vi "GE 5565PIORC.Memory.Deallocate Block.vi"(8 "error in (no error)":errorcluster, 10 "Block Descriptor":T1 {"next descriptor ptr" format="%08x"; "data size" format="%08x"; "data ptr (upper)" format="%08x"; "data ptr (lower)" format="%08x"; "descriptor ptr (aligned)" format="%08x"; "descriptor size" format="%08x"; "descriptor ptr (VISA)" format="%08x"}, 11 "GE 5565PIORC in":refnum<class "GE 5565PIORC.lvclass">) -> (0 "error out":errorcluster, 3 "GE 5565PIORC out":refnum<class "GE 5565PIORC.lvclass">)   [LabVIEW 2016, in "GE 5565PIORC.lvclass"]
uses:
  GE 5565PIORC.lvclass
  Typedefs/GE 5565PIORC.Typdef.DMA Block Descriptor.ctl
  GE 5565PIORC.lvclass/GE 5565PIORC.ctl
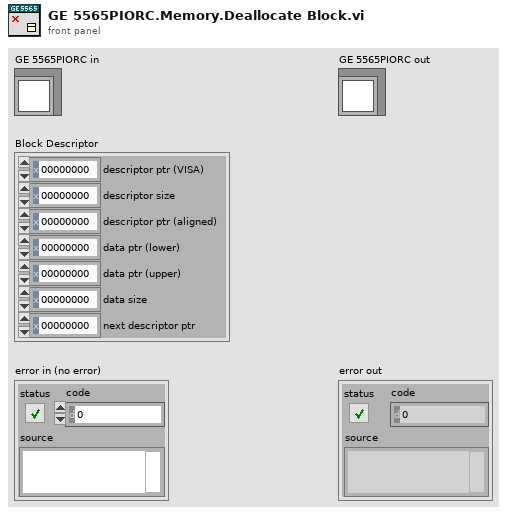
[diagram p1: front panel]
types:
  T1 = typedef "GE 5565PIORC.lvclass/GE 5565PIORC.Typdef.DMA Block Descriptor.ctl" = cluster{"descriptor ptr (VISA)":u32, "descriptor size":u32, "descriptor ptr (aligned)":u32, "data ptr (lower)":u32, "data ptr (upper)":u32, "data size":u32, "next descriptor ptr":u32}
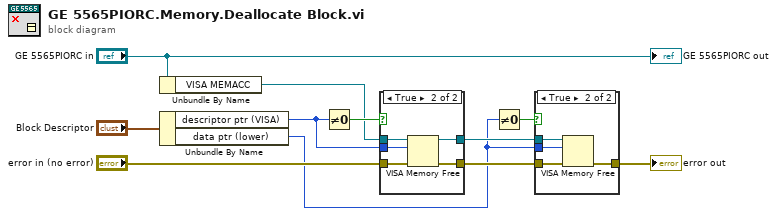
[diagram p0: block diagram]
diagram:
  n1 = Unbundle By Name("GE 5565PIORC in") -> ("VISA MEMACC"=w9:refnum<visa-resource-name>)
  n2 = Unbundle By Name("Block Descriptor") -> ("descriptor ptr (VISA)"=w11:u32, "data ptr (lower)"=w1:u32)
  n3 = Not Equal To 0?(x=w11) -> (x != 0?=w10:bool)
  n4 = case shown="True" w10 {
    tunnel: "error in (no error)" -> [w13 w18]
    tunnel: [w13 w17] -> w8
    tunnel: w9 -> [w12 w16]
    tunnel: w11 -> [_ w15]
    tunnel: [w12 w14] -> w7
    frame False {
    }
    frame True {
      n5 = VISA Memory Free(8:w18, 10:w15, 11:w16) -> (0:w17:errorcluster, 3:w14:refnum<visa-resource-name>)
    }
  }
  n6 = Not Equal To 0?(x=w1) -> (x != 0?=w6:bool)
  n7 = case shown="True" w6 {
    tunnel: w8 -> [w19 w23]
    tunnel: [w19 w22] -> w4
    tunnel: w7 -> [_ w21]
    tunnel: w1 -> [_ w20]
    frame False {
    }
    frame True {
      n8 = VISA Memory Free(8:w23, 10:w20, 11:w21) -> (0:w22:errorcluster)  [unwired: 1 out]
    }
  }
  "error out" <- w4
  "GE 5565PIORC out" <- "GE 5565PIORC in"
